vi "Word_Color_to_RGB.vi"(0 "word color table index":i32) -> (1 "R":u8, 2 "G":u8, 3 "B":u8)   [LabVIEW 2020, in "NI_ReportGenerationToolkit.lvlib"]
uses:
  <vilib>/addons/_office/NI_ReportGenerationToolkit.lvlib
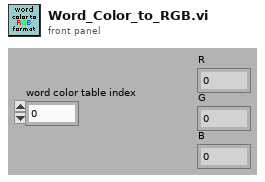
[diagram p1: front panel]
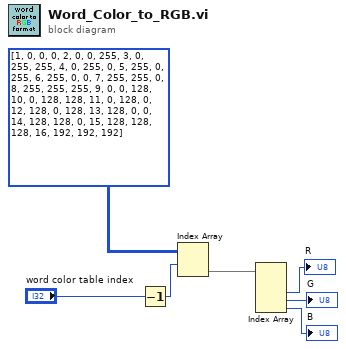
[diagram p0: block diagram]
diagram:
  n1 = Decrement(x="word color table index") -> (x-1=w6:i32)
  n2 = Index Array(array=i32[][] [[1, 0, 0, 0], [2, 0, 0, 255], [3, 0, 255, 255], [4, 0, 255, 0], [5, 255, 0, 255], [6, 255, 0, 0], [7, 255, 255, 0], [8, 255, 255, 255], [9, 0, 0, 128], [10, 0, 128, 128], [11, 0, 128, 0], [12, 128, 0, 128], [13, 128, 0, 0], [14, 128, 128, 0], [15, 128, 128, 128], [16, 192, 192, 192]] ("data"), index (row)=w6) -> (element=w5:i32[])  [unwired: 1 in]
  n3 = Index Array(array=w5) -> (element #2=→"R":i32, element #3=→"G":i32, element #4=→"B":i32)  [unwired: 4 in, 1 out]
